vi "K-Means.vi"(6 "stopping criteria":cluster{"tolarence":dbl, "max iterations":i32}={"tolarence"=1e-05, "max iterations"=50}, 8 "error in (no error)":errorcluster, 9 "# of classes":i32=1, 10 "Centroids (initial)":dbl[][](array[numeric]), 11 "Data samples":dbl[][](array[numeric])) -> (0 "error out":errorcluster, 2 "Centroids":dbl[][](array[numeric]), 3 "Class labels":i32[](array[numeric]))   [LabVIEW 2013, in "NILabs_MLT.lvlib"]
uses:
  <vilib>/addons/Machine Learning/NILabs_MLT.lvlib
  <vilib>/Analysis/_algsub.llb/Matrix Norm Type.ctl
  <vilib>/Analysis/_algsub.llb/Real Matrix Norm.vi
  <vilib>/Analysis/NI_AALPro.lvlib
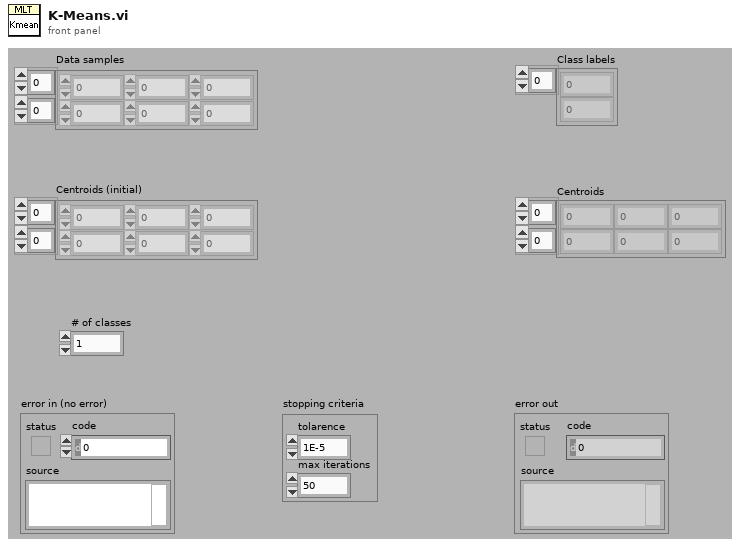
[diagram p1: front panel]
types:
  T1 = typedef "NI_AALPro.lvlib/Matrix Norm Type.ctl" = i32
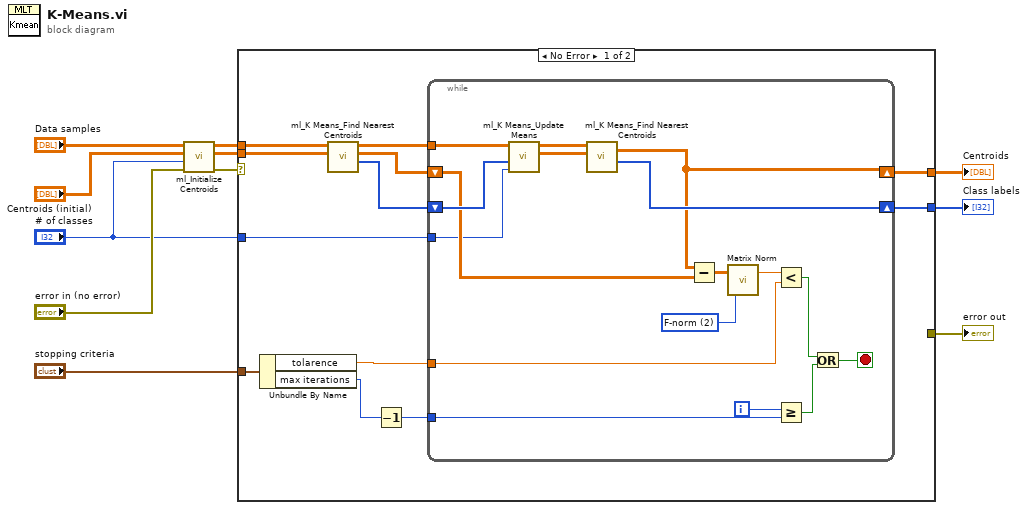
[diagram p0: block diagram]
diagram:
  n1 = call <vilib>:"ml_Initialize Centroids.vi"("error in (no error)"="error in (no error)", "# of classes"="# of classes", "Centroids in"="Centroids (initial)", "Samples"="Data samples") -> ("error out"=w3:errorcluster, "Centroids out"=w10:dbl[][], "Samples dup"=w11:dbl[][])  [unwired: 5 in]
  n2 = case shown="No Error" w3 {
    selector: w3 -> [_ w41]
    tunnel: w11 -> [w23 _]
    tunnel: w10 -> [w22 _]
    tunnel: [w18 _] -> w6
    tunnel: [w17 _] -> w5
    tunnel: "# of classes" -> [w15 _]
    tunnel: [_ w41] -> w2
    tunnel: "stopping criteria" -> [w14 _]
    frame No Error {
      n3 = Unbundle By Name(w14) -> ("tolarence"=w13:dbl, "max iterations"=w12:i32)
      n4 = call <vilib>:"ml_K Means_Find Nearest Centroids.vi"("Centroids"=w22, "Samples"=w23) -> ("nearest centroid"=w19:i32[], "Centroids dup"=w20:dbl[][], "Samples dup"=w21:dbl[][])  [unwired: 7 in]
      n5 = Decrement(x=w12) -> (x-1=w16:i32)
      n6 = while {
        tunnel: w21 -> [w40]
        shift-right: [w33] -> w17
        shift-left: w20 -> [w32]
        shift-right: [w36] -> w18
        shift-left: w19 -> [w39]
        tunnel: w13 -> [w28]
        tunnel: w16 -> [w29]
        tunnel: w15 -> [w24]
        i -> [w30]
        stop <- w25 stop-if-true
        w31 = T1 2 items=["2-norm", "1-norm", "F-norm", "Inf-norm"] ("norm type")
        n7 = call <vilib>:"ml_K Means_Update Means.vi"("# of classes"=w24, "labels"=w39, "Samples"=w40) -> ("Means"=w37:dbl[][], "Samples dup"=w38:dbl[][])  [unwired: 5 in, 2 out]
        n8 = call <vilib>:"ml_K Means_Find Nearest Centroids.vi"("Centroids"=w37, "Samples"=w38) -> ("nearest centroid"=w36:i32[], "Centroids dup"=w33:dbl[][])  [unwired: 7 in, 1 out]
        n9 = Subtract ("Subtract.vi")(x=w33, y=w32) -> (x-y=w35:dbl[][])
        n10 = call-poly <vilib>:"Matrix Norm.vi"("norm type"=w31, "Input Matrix"=w35) -> ("norm"=w34:dbl)  [unwired: 1 out]
        n11 = Less?(x=w34, y=w28) -> (x < y?=w27:bool)
        n12 = Greater Or Equal?(x=w30, y=w29) -> (x >= y?=w26:bool)
        n13 = Or(x=w27, y=w26) -> (x .or. y?=w25:bool)
      }
    }
    frame Error {
    }
  }
  "Class labels" <- w6
  "Centroids" <- w5
  "error out" <- w2
